vi "EvaluaParoEmergencia.vi"(0 "EsticPujant":bool, 5 "FCI":bool, 7 "FCS":bool, 9 "EsticBaixant":bool, 11 "ParoManual":bool) -> (6 "Paro":bool)   [LabVIEW 2017]
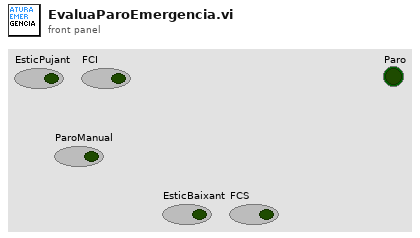
[diagram p1: front panel]
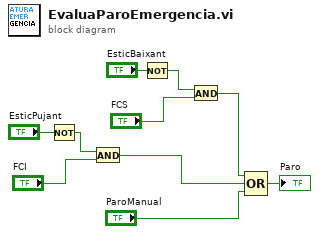
[diagram p0: block diagram]
diagram:
  n1 = Not(x="EsticPujant") -> (.not. x?=w5:bool)
  n2 = And(x=w5, y="FCI") -> (x .and. y?=w4:bool)
  n3 = Not(x="EsticBaixant") -> (.not. x?=w3:bool)
  n4 = And(x=w3, y="FCS") -> (x .and. y?=w2:bool)
  n5 = Compound Arithmetic op=OR(w2, w4, "ParoManual") -> (→"Paro":bool)
